vi "DIM_Read Latest Data.vi"(8 "error in (no error)":errorcluster, 10 "Src.SysLabels":string[](array[string]), 11 "UI_Actor in":refnum<class "UI_Actor.lvclass">) -> (0 "error out":errorcluster, 2 "Latest Data":dbl[](array[numeric]), 3 "UI_Actor out":refnum<class "UI_Actor.lvclass">)   [LabVIEW 2020, in "UI_Actor.lvlib" / "UI_Actor.lvclass"]
uses:
  UI_Actor.lvclass
  UI_Actor.lvclass/UI_Actor.ctl
  support/Databox.lvlibp/TypesTools/Config/Config.lvclass
  support/Databox.lvlibp/TypesTools/Data/Data.lvclass
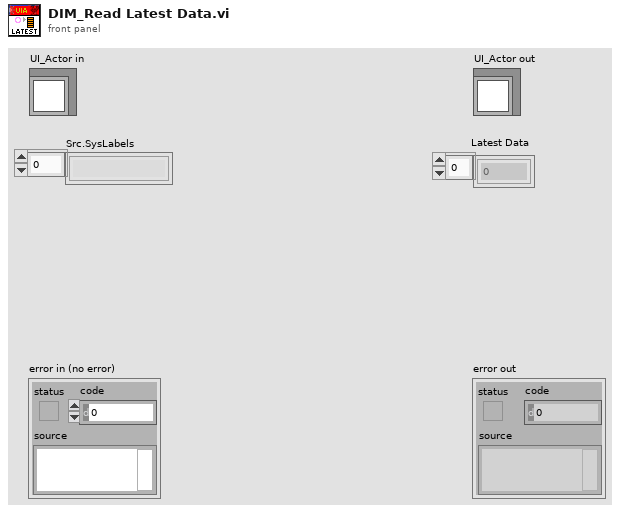
[diagram p1: front panel]
types:
  T1 = typedef "UI_Actor.lvlib/UI_Actor.lvclass/ctl_InternalMapItem.ctl" = cluster{"Config":refnum<class "Config.lvclass">, "LatestData":refnum<class "Data.lvclass">}
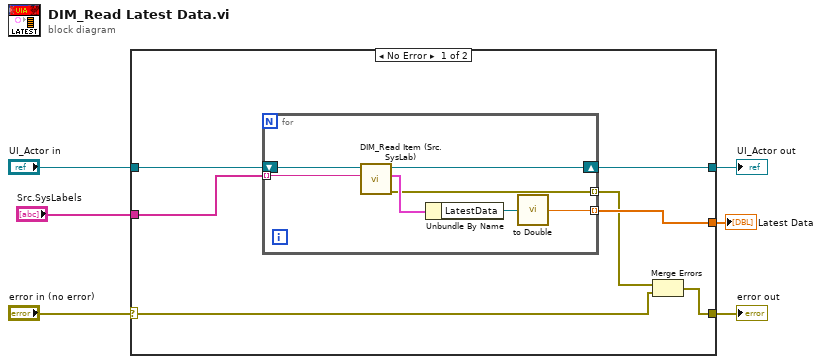
[diagram p0: block diagram]
diagram:
  n1 = case shown="No Error" "error in (no error)" {
    selector: "error in (no error)" -> [w13 w22]
    tunnel: [w12 w22] -> w5
    tunnel: [w10 w21] -> w3
    tunnel: "UI_Actor in" -> [w9 w21]
    tunnel: [w8 _] -> w2
    tunnel: "Src.SysLabels" -> [w11 _]
    frame No Error {
      n2 = for {
        tunnel: w11 -> [w20] mode=indexing
        tunnel: [w15] -> w8 mode=indexing
        shift-right: [w19] -> w10
        shift-left: w9 -> [w18]
        tunnel: [w14] -> w7 mode=indexing
        n3 = call "DIM_Read Item (Src.SysLab).vi"("Sourcer.SysLabel"=w20, "UI_Actor in"=w18) -> ("error out"=w14:errorcluster, "DIM Item"=w17:T1, "UI_Actor out"=w19:refnum<class "UI_Actor.lvclass">)  [unwired: 6 in, 1 out]
        n4 = Unbundle By Name(w17) -> ("LatestData"=w16:refnum<class "Data.lvclass">)
        n5 = call "to Double.vi"("Data"=w16) -> ("Double"=w15:dbl)
      }
      n6 = Merge Errors(w7, w13) -> (w12:errorcluster)
    }
    frame Error {
    }
  }
  "error out" <- w5
  "UI_Actor out" <- w3
  "Latest Data" <- w2
